vi "Read Configuration Parameters.vi"(8 "error in (no error)":errorcluster, 10 "refnum":T1, 11 "CCD Configuration in":refnum<class "CCD Configuration.lvclass">) -> (0 "error out":errorcluster, 2 "refnum out":T1, 3 "CCD Configuration out":refnum<class "CCD Configuration.lvclass">)   [LabVIEW 2016, in "CCD.lvlib" / "CCD Configuration.lvclass"]
uses:
  <userlib>/Common Components/Hardware/CCD/CCD Configuration.lvclass
  <vilib>/Utility/config.llb/Config Data RefNum.ctl
  <userlib>/Common Components/Hardware/CCD/CCD Configuration.lvclass/CCD Configuration.ctl
  <userlib>/Common Components/Hardware/Abstract Hardware/Hardware.lvclass/Hardware.ctl
  <userlib>/Common Components/Hardware/CCD/CCD/CCD.lvclass/CCD.ctl
  <userlib>/Common Components/Hardware/CCD/CCD Configuration/Write Hardware.lvlib_CCD.lvlib_CCD.lvclass.vi
  <userlib>/Common Components/Hardware/CCD/CCD Configuration/Read Hardware.lvlib_CCD.lvlib_CCD.lvclass.vi
  <userlib>/Common Components/Hardware/Abstract Hardware/Read Label.vi
  <userlib>/Common Components/Hardware/CCD/CCD/CCD.lvclass
  C:/Program Files (x86)/National Instruments/LabVIEW 2016/user.lib/Common Components/Hardware/Abstract Hardware/Hardware.lvclass
  <vilib>/Utility/config.llb/NI_LVConfig.lvlib
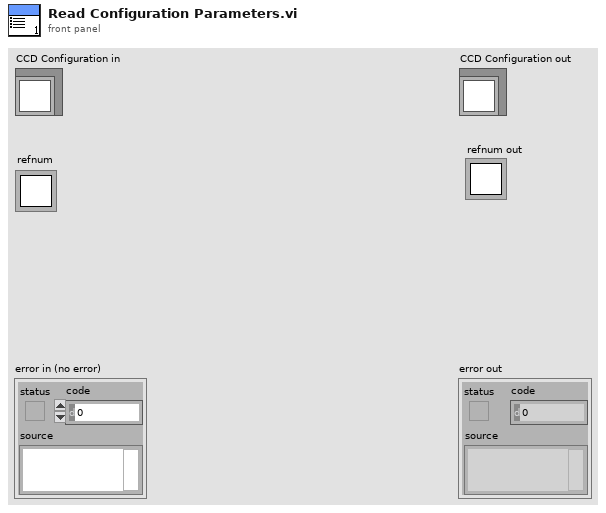
[diagram p1: front panel]
types:
  T1 = typedef "NI_LVConfig.lvlib/Config Data RefNum.ctl" = refnum<k1>
  T2 = typedef "CCD.lvlib/CCD.lvclass/camer data.ctl" = cluster{"VideoMode":u16, "gain":u32, "gamma":sgl, "Contrast":dbl, "Exposure":u32, "Saturation":u32}
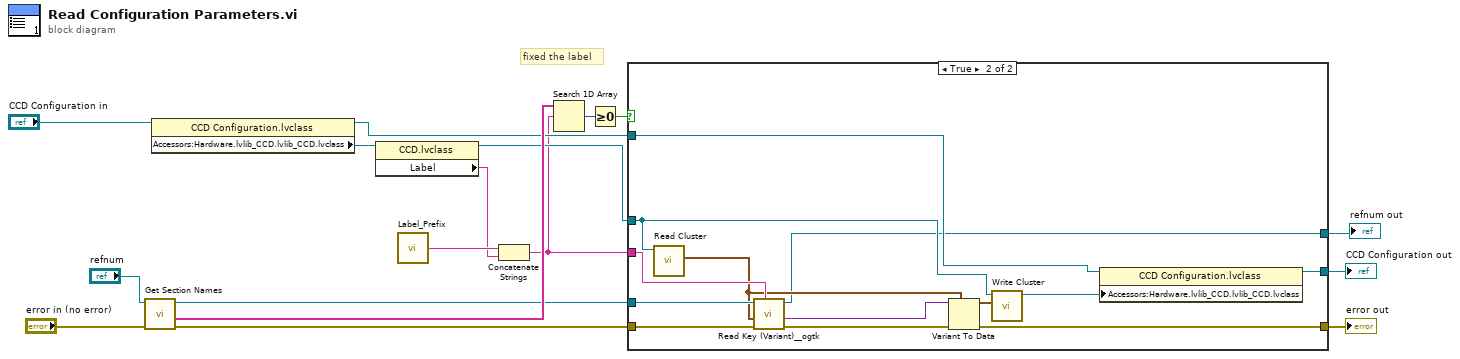
[diagram p0: block diagram]
diagram:
  # "fixed the label"
  n1 = call <vilib>:"Get Section Names.vi"("error in (no error)"="error in (no error)", "refnum"="refnum") -> ("error out"=w6:errorcluster, "section names"=w11:string[], "refnum out"=w7:T1)  [unwired: 7 in]
  n2 = property class="CCD Configuration.lvclass"(reference="CCD Configuration in") -> (reference out=w8:refnum<class "CCD Configuration.lvclass">, "Accessors:Hardware.lvlib_CCD.lvlib_CCD.lvclass"=w13:refnum<class "CCD.lvclass">)  [unwired: 1 in, 1 out]
  n3 = property class="CCD.lvclass"(reference=w13) -> (reference out=w5:refnum<class "CCD.lvclass">, "Label"=w12:string)  [unwired: 1 in, 1 out]
  n4 = call <userlib>:"Label_Prefix.vi"() -> ("Label Prefix String"=w14:string)
  n5 = Concatenate Strings(w14, w12) -> (w1:string)
  n6 = Search 1D Array(1D array=w11, element=w1) -> (index of element=w10:i32)  [unwired: 1 in]
  n7 = Greater Or Equal To 0?(x=w10) -> (x >= 0?=w9:bool)
  n8 = case shown="True" w9 {
    tunnel: w8 -> [w20 w25]
    tunnel: w7 -> [w19 w33]
    tunnel: w6 -> [w18 w23]
    tunnel: w5 -> [_ w28]
    tunnel: [w20 w26] -> w4
    tunnel: [w19 w24] -> w3
    tunnel: [w18 w21] -> w2
    tunnel: w1 -> [_ w32]
    frame False {
    }
    frame True {
      n9 = call <userlib>:"Read Cluster.vi"("CCD in"=w28) -> ("Cluster"=w30:T2)  [unwired: 8 in, 2 out]
      n10 = call <userlib>:"Read Key (Variant)__ogtk.vi"("section"=w32, "error in (no error)"=w23, "type"=w30, "refnum"=w33) -> ("error out"=w22:errorcluster, "key-value"=w31:variant, "refnum out"=w24:T1)  [unwired: 4 in, 1 out]
      n11 = Variant To Data(error in=w22, type=w30, Variant=w31) -> (data=w29:T2, error out=w21:errorcluster)
      n12 = call <userlib>:"Write Cluster.vi"("Cluster"=w29, "CCD in"=w28) -> ("CCD out"=w27:refnum<class "CCD.lvclass">)  [unwired: 8 in, 1 out]
      n13 = property class="CCD Configuration.lvclass"(reference=w25, "Accessors:Hardware.lvlib_CCD.lvlib_CCD.lvclass"=w27) -> (reference out=w26:refnum<class "CCD Configuration.lvclass">)  [unwired: 1 in, 1 out]
    }
  }
  "error out" <- w2
  "CCD Configuration out" <- w4
  "refnum out" <- w3
